vi "读写字符串DEMO.vi"() -> ()   [LabVIEW 2012]
panel:
  out "字符串":string
  in  "停止":bool
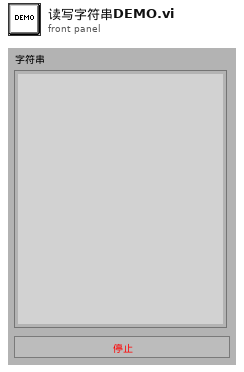
[diagram p1: front panel]
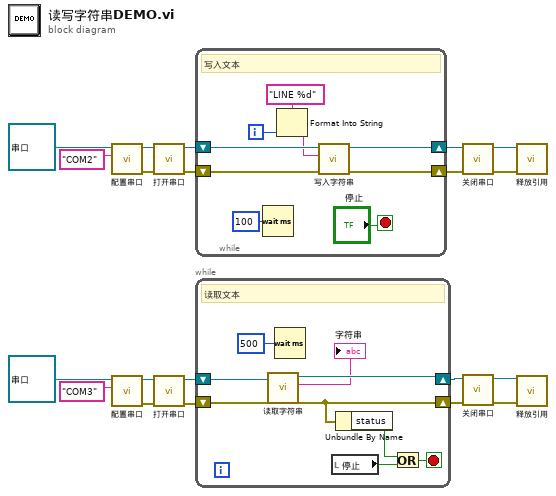
[diagram p0: block diagram]
diagram:
  n1 = call "配置串口.vi"("Port Name"="COM2", "COM 输入"=refnum<class "串口.lvclass"> refnum ("串口.lvclass")) -> ("error out"=w17:errorcluster, "COM 输出"=w18:refnum<class "串口.lvclass">)  [unwired: 8 in]
  n2 = call "配置串口.vi"("Port Name"="COM3", "COM 输入"=refnum<class "串口.lvclass"> refnum ("串口.lvclass")) -> ("error out"=w1:errorcluster, "COM 输出"=w2:refnum<class "串口.lvclass">)  [unwired: 8 in]
  n3 = call "打开串口.vi"("error in (no error)"=w17, "串口 输入"=w18) -> ("error out"=w15:errorcluster, "串口 输出"=w16:refnum<class "串口.lvclass">)  [unwired: 8 in]
  n4 = call "打开串口.vi"("error in (no error)"=w1, "串口 输入"=w2) -> ("error out"=w5:errorcluster, "串口 输出"=w6:refnum<class "串口.lvclass">)  [unwired: 8 in]
  n5 = while {
    shift-right: [w21] -> w13
    shift-left: w15 -> [w24]
    shift-right: [w22] -> w14
    shift-left: w16 -> [w25]
    i -> [w28]
    stop <- "停止" stop-if-true
    # "写入文本"
    n6 = Wait (ms)(milliseconds to wait=u32 100 ("等待时间（毫秒）")) -> ()  [unwired: 1 out]
    n7 = Format Into String(format string="LINE %d" ("格式字符串"), w28) -> (resulting string=w23:string)  [unwired: 2 in, 1 out]
    n8 = call "写入字符串.vi"("error in (no error)"=w24, "字符串"=w23, "串口 输入"=w25) -> ("error out"=w21:errorcluster, "串口 输出"=w22:refnum<class "串口.lvclass">)  [unwired: 7 in]
  }
  n9 = while {
    shift-right: [w33] -> w4
    shift-left: w5 -> [w37]
    shift-right: [w35] -> w3
    shift-left: w6 -> [w36]
    stop <- w30 stop-if-true
    # "读取文本"
    n10 = call "读取字符串.vi"("error in (no error)"=w37, "串口 输入"=w36) -> ("error out"=w33:errorcluster, "字符串"=→"字符串":string, "串口 输出"=w35:refnum<class "串口.lvclass">)  [unwired: 7 in]
    n11 = Wait (ms)(milliseconds to wait=u32 500 ("等待时间（毫秒）")) -> ()  [unwired: 1 out]
    n12 = local read "停止"() -> (w31:bool)
    n13 = Unbundle By Name(w33) -> ("status"=w32:bool)
    n14 = Or(x=w32, y=w31) -> (x .or. y?=w30:bool)
  }
  n15 = call "关闭串口.vi"("error in (no error)"=w13, "串口 输入"=w14) -> ("error out"=w12:errorcluster, "串口 输出"=w11:refnum<class "串口.lvclass">)  [unwired: 8 in]
  n16 = call "关闭串口.vi"("error in (no error)"=w4, "串口 输入"=w3) -> ("error out"=w7:errorcluster, "串口 输出"=w8:refnum<class "串口.lvclass">)  [unwired: 8 in]
  n17 = call "释放引用.vi"("error in (no error)"=w12, "串口 输入"=w11) -> ()  [unwired: 8 in, 2 out]
  n18 = call "释放引用.vi"("error in (no error)"=w7, "串口 输入"=w8) -> ()  [unwired: 8 in, 2 out]
